vi "Create Table.vi"(8 "error in (no error)":errorcluster, 10 "SQL Statement":string="CREATE TABLE IF NOT EXISTS Sensors (\n    SensorID INTEGER PRIMARY KEY AUTOINCREMENT,\n    SerialNumber TEXT UNIQUE NOT NULL,\n    ModelNumber TEXT NOT NULL,\n    Min REAL NOT NULL,\n    Max REAL NOT NULL,\n    Units TEXT NOT NULL,\n    OutputSignal TEXT NOT NULL,\n    created_at DATETIME DEFAULT CURRENT_TIMESTAMP\n);", 11 "Refnum in":T1) -> (0 "error out":errorcluster, 3 "Refnum out":T1)   [LabVIEW 2026, in "Database.lvlib"]
uses:
  Database.lvlib
  <vilib>/addons/database/NI_Database_API.lvlib
  <vilib>/addons/database/Connection.llb/Conn Execute.vi
  <vilib>/addons/database/Recordset.llb/Rec Destroy - Connection.vi
  <vilib>/addons/database/Connection.llb/Conn ObjectReference.ctl
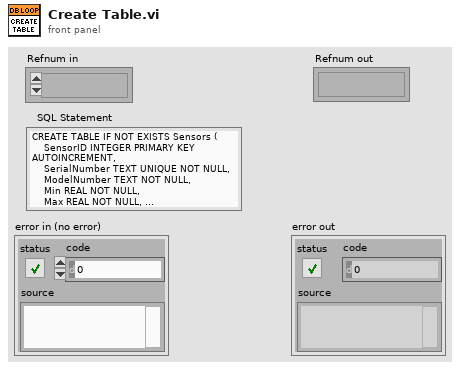
[diagram p1: front panel]
types:
  T1 = typedef "NI_Database_API.lvlib/Conn ObjectReference.ctl" = refnum<k1>
  T2 = typedef "NI_Database_API.lvlib/Rec ObjectReference.ctl" = refnum<k1>
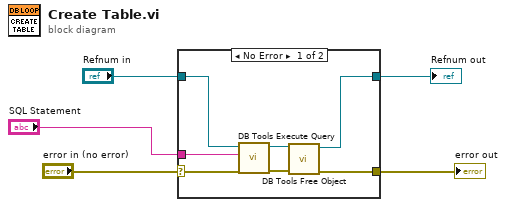
[diagram p0: block diagram]
diagram:
  n1 = case shown="No Error" "error in (no error)" {
    selector: "error in (no error)" -> [w6 w14]
    tunnel: "Refnum in" -> [w12 w13]
    tunnel: [w11 w13] -> w4
    tunnel: [w10 w14] -> w3
    tunnel: "SQL Statement" -> [w9 _]
    frame No Error {
      n2 = call-poly <vilib>:"DB Tools Execute Query.vi"("error in (no error)"=w6, "SQL query"=w9, "connection reference"=w12) -> ("error out"=w7:errorcluster, "recordset reference"=w8:T2)  [unwired: 5 in]
      n3 = call-poly <vilib>:"DB Tools Free Object.vi"("error in (no error)"=w7, "recordset reference"=w8) -> ("error out"=w10:errorcluster, "connection reference"=w11:T1)  [unwired: 8 in]
    }
    frame Error {
    }
  }
  "Refnum out" <- w4
  "error out" <- w3
